vi "dmd_period_count_sub.vi"() -> ()   [LabVIEW 2020]
uses:
  <vilib>/Utility/error.llb/DialogType.ctl
  <vilib>/DAQmx/read.llb/DAQmx Read (Counter 1D U32 1Chan NSamp).vi
  <vilib>/DAQmx/create/channels.llb/DAQmx Create Channel (CI-Period).vi
  <vilib>/DAQmx/create/channels.llb/DAQmx Create Channel (CO-Pulse Generation-Frequency).vi
  <vilib>/DAQmx/configure/timing.llb/DAQmx Timing (Implicit).vi
  <vilib>/DAQmx/miscellaneous.llb/DAQmx Fill In Error Info.vi
  <resource>/objmgr/daqmx.rc
panel:
  out "Loop Time (ms) 2":u32=10
  out "data":u32[](graph)
  out "Input.BufSize":u32=1000000 format="%.0p"
  out "Consumer Iteration 2":i32=1109257
  in  "stop 3":bool
  in  "number of samples per channel 2":i32=5000
  out "Producer Iteration 2":i32=1109256
  out "error out 2":errorcluster
  in  "dwell time (ms)":dbl=1.0 format="%.6f"
  in  "Photon Input (PFI)":tag="/Dev1/PFI0"
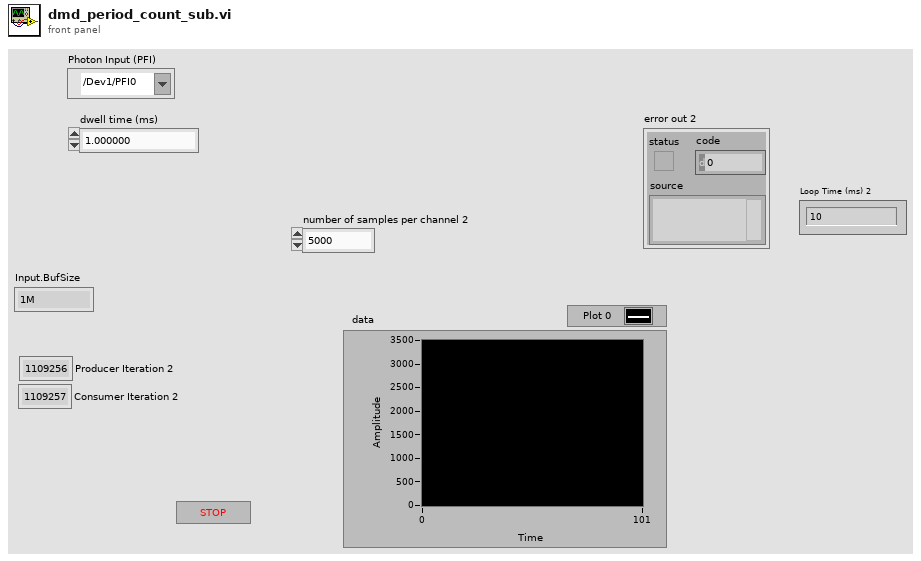
[diagram p1: front panel]
types:
  T1 = enum16{"open", "open or create", "create or replace", "create", "open (read-only)"}
  T2 = typedef "DialogType.ctl" = u16
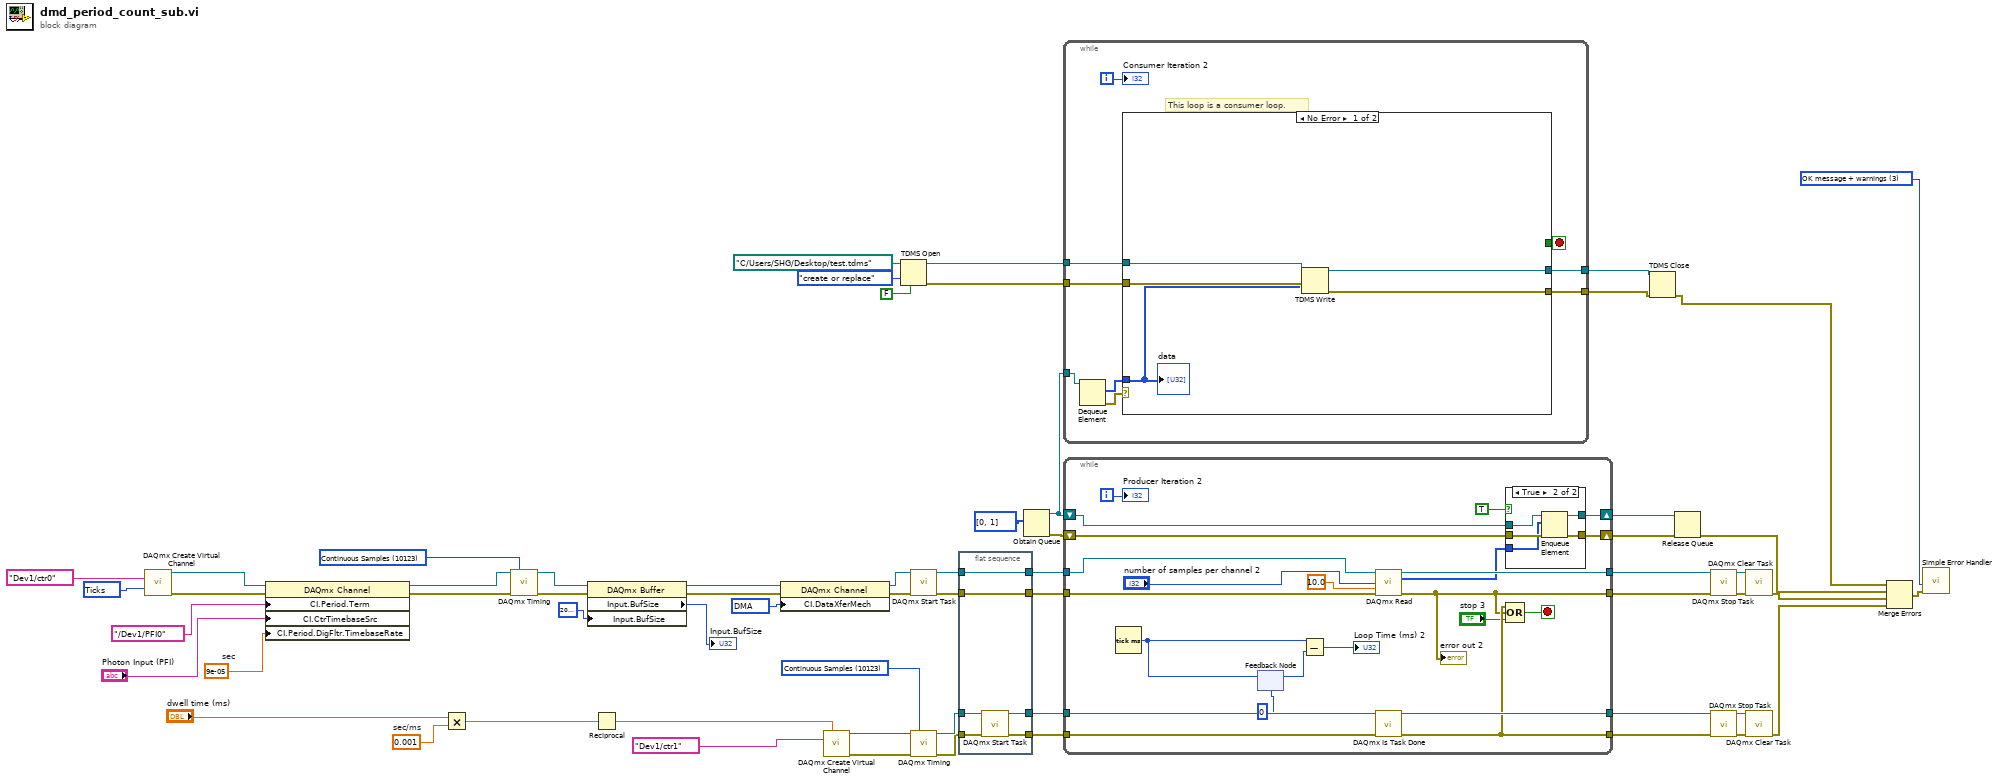
[diagram p0: block diagram]
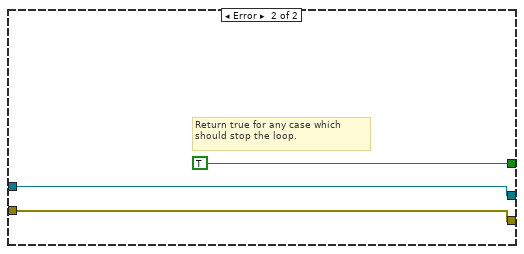
[diagram p2: hidden frame]
diagram:
  w10 = T2 3 items=["no dialog", "OK message", "continue or stop message", "OK message + warnings", "continue/stop + warnings"] ("type of dialog (OK msg:1)")
  w1 = 9e-05  # sec
  w23 = 10054 items=["DMA"=10054, "Interrupts"=10204, "Programmed I/O"=10264, "USB Bulk"=12590] ("CI.DataXferMech")
  w43 = 0.001  # sec/ms
  w53 = 10304 items=["Seconds"=10364, "Ticks"=10304, "From Custom Scale"=10065] ("units")
  w54 = 10123 items=["Finite Samples"=10178, "Continuous Samples"=10123, "Hardware Timed Single Point"=12522] ("sample mode")
  w55 = 10123 items=["Finite Samples"=10178, "Continuous Samples"=10123, "Hardware Timed Single Point"=12522] ("sample mode")
  n1 = call-poly <vilib>:"DAQmx Create Virtual Channel.vi"("counter"=tag "Dev1/ctr0", "units"=w53) -> ("task out"=w50:refnum<k21>, "error out"=w49:errorcluster)  [unwired: 12 in]
  n2 = property class="DAQmx Channel"(reference=w50, error in=w49, "CI.Period.Term"=tag "/Dev1/PFI0", "CI.CtrTimebaseSrc"="Photon Input (PFI)", "CI.Period.DigFltr.TimebaseRate"=w1) -> (reference out=w48:refnum<k21>, error out=w47:errorcluster)
  n3 = Multiply(x="dwell time (ms)", y=w43) -> (x*y=w42:dbl)
  n4 = call-poly <vilib>:"DAQmx Timing.vi"("task/channels in"=w48, "sample mode"=w54, "error in"=w47) -> ("task out"=w18:refnum<k21>, "error out"=w17:errorcluster)  [unwired: 11 in]
  n5 = property class="DAQmx Buffer"(reference=w18, error in=w17, "Input.BufSize"=u32 2000000 ("samples per channel")) -> (reference out=w22:refnum<k21>, error out=w20:errorcluster, "Input.BufSize"=→"Input.BufSize":u32)
  n6 = Reciprocal(x=w42) -> (1/x=w41:dbl)
  n7 = property class="DAQmx Channel"(reference=w22, error in=w20, "CI.DataXferMech"=w23) -> (reference out=w16:refnum<k21>, error out=w15:errorcluster)
  n8 = call-poly <vilib>:"DAQmx Create Virtual Channel.vi"("frequency"=w41, "counter"=tag "Dev1/ctr1") -> ("task out"=w60:refnum<k21>, "error out"=w61:errorcluster)  [unwired: 12 in]
  n9 = TDMS Open(6:FALSE ("disable buffering? (T)"), 10:T1."create or replace" ("operation (0:open)"), 11:path "C:/Users/SHG/Desktop/test.tdms" ("file path")) -> (0:w12:errorcluster, 3:w14:refnum<k34>)  [unwired: 4 in]
  n10 = call <vilib>:"DAQmx Start Task.vi"("task/channels in"=w16, "error in"=w15) -> ("task out"=w40:refnum<k21>, "error out"=w39:errorcluster)  [unwired: 12 in]
  n11 = call-poly <vilib>:"DAQmx Timing.vi"("task/channels in"=w60, "sample mode"=w55, "error in"=w61) -> ("task out"=w59:refnum<k21>, "error out"=w58:errorcluster)  [unwired: 11 in]
  n12 = flat-sequence {
    tunnel: w59 -> [w67]
    tunnel: w58 -> [w66]
    tunnel: [w65] -> w26
    tunnel: [w64] -> w27
    tunnel: w40 -> [w62]
    tunnel: w39 -> [w63]
    tunnel: [w63] -> w29
    tunnel: [w62] -> w28
    frame #0 {
      n13 = call <vilib>:"DAQmx Start Task.vi"("task/channels in"=w67, "error in"=w66) -> ("task out"=w64:refnum<k21>, "error out"=w65:errorcluster)  [unwired: 12 in]
    }
  }
  n14 = Obtain Queue(element data type=u32[] [0, 1] ("data")) -> (queue out=w38:refnum<queue>, error out=w37:errorcluster)  [unwired: 4 in, 1 out]
  n15 = while {
    tunnel: w38 -> [w76]
    tunnel: w14 -> [w71]
    tunnel: [w70] -> w13
    tunnel: w12 -> [w69]
    tunnel: [w68] -> w11
    i -> [w72]
    stop <- w73 stop-if-true
    # "This loop is a consumer loop."
    n16 = Dequeue Element(queue=w76) -> (element=w74:u32[], error out=w75:errorcluster)  [unwired: 2 in, 2 out]
    n17 = case shown="No Error" w75 {
      tunnel: w74 -> [w77 _]
      tunnel: [_ TRUE] -> w73
      tunnel: w71 -> [w81 w83]
      tunnel: [w80 w83] -> w70
      tunnel: w69 -> [w79 w82]
      tunnel: [w78 w82] -> w68
      frame No Error {
        n18 = TDMS Write(0:w81, 9:w77, 11:w79) -> (4:w80:refnum<k34>, 15:w78:errorcluster)  [unwired: 3 in, 2 out]
        "data" <- w77
      }
      frame Error {
        # "Return true for any case which should stop the loop."
      }
    }
    "Consumer Iteration 2" <- w72
  }
  n19 = while {
    shift-right: [w96] -> w35
    shift-left: w37 -> [w105]
    shift-right: [w106] -> w36
    shift-left: w38 -> [w107]
    tunnel: [w103] -> w32
    tunnel: [w91] -> w31
    tunnel: w29 -> [w102]
    tunnel: w28 -> [w101]
    tunnel: w27 -> [w95]
    tunnel: w26 -> [w94]
    tunnel: [w93] -> w25
    tunnel: [w92] -> w24
    i -> [w97]
    stop <- w89 stop-if-true
    n20 = Tick Count (ms)() -> (millisecond timer value=w88:u32)
    n21 = feedback #1(u32 0 ("millisecond timer value")) -> (w87:u32)
    n22 = feedback-in #1(w88) -> ()
    n23 = Subtract(x=w88, y=w87) -> (x-y=→"Loop Time (ms) 2":u32)
    n24 = call-poly <vilib>:"DAQmx Read.vi"("task/channels in"=w101, "number of samples per channel"="number of samples per channel 2", "timeout"=10.0, "error in"=w102) -> ("task out"=w103:refnum<k21>, "data"=w100:u32[], "error out"=w91:errorcluster)  [unwired: 9 in]
    "error out 2" <- w91
    n25 = call <vilib>:"DAQmx Is Task Done.vi"("task/channels in"=w95, "error in"=w94) -> ("task out"=w93:refnum<k21>, "error out"=w92:errorcluster)  [unwired: 11 in, 1 out]
    n26 = case shown="True" TRUE ("Case Constant\n(See Context Help)") {
      tunnel: w107 -> [w109 w114]
      tunnel: [w109 w113] -> w106
      tunnel: w105 -> [w108 w112]
      tunnel: [w108 w111] -> w96
      tunnel: w100 -> [_ w110]
      frame False {
      }
      frame True {
        n27 = Enqueue Element(queue=w114, element=w110, error in (no error)=w112) -> (queue out=w113:refnum<queue>, error out=w111:errorcluster)  [unwired: 1 in, 1 out]
      }
    }
    n28 = Compound Arithmetic op=OR(w92, w91, "stop 3") -> (w89:bool)
    "Producer Iteration 2" <- w97
  }
  n29 = TDMS Close(8:w11, 11:w13) -> (0:w6:errorcluster)  [unwired: 1 out]
  n30 = Release Queue(queue=w36, error in (no error)=w35) -> (error out=w5:errorcluster)  [unwired: 1 in, 2 out]
  n31 = call <vilib>:"DAQmx Stop Task.vi"("task/channels in"=w32, "error in"=w31) -> ("task out"=w33:refnum<k21>, "error out"=w34:errorcluster)  [unwired: 12 in]
  n32 = call <vilib>:"DAQmx Stop Task.vi"("task/channels in"=w25, "error in"=w24) -> ("task out"=w57:refnum<k21>, "error out"=w56:errorcluster)  [unwired: 12 in]
  n33 = call <vilib>:"DAQmx Clear Task.vi"("task in"=w33, "error in"=w34) -> ("error out"=w4:errorcluster)  [unwired: 13 in]
  n34 = call <vilib>:"DAQmx Clear Task.vi"("task in"=w57, "error in"=w56) -> ("error out"=w3:errorcluster)  [unwired: 13 in]
  n35 = Merge Errors(w6, w5, w4, w3) -> (w9:errorcluster)
  n36 = call <vilib>:"Simple Error Handler.vi"("type of dialog (OK msg:1)"=w10, "error in (no error)"=w9) -> ()  [unwired: 3 in, 5 out]
